vi "Read Module Configuration from Switches JSON.vi"(8 "error in":errorcluster, 11 "switches json file":path) -> (0 "error out":errorcluster, 2 "switches json":string, 3 "topologies":string[](array[string]))   [LabVIEW 2020, in "SLSC Switch Scripting.lvlib"]
uses:
  SLSC Switch Scripting.lvlib
  <vilib>/SLSC_Switch/Get Topologies (Simulate).vi
  <vilib>/SLSC_Switch/SLSC Switch.lvlib
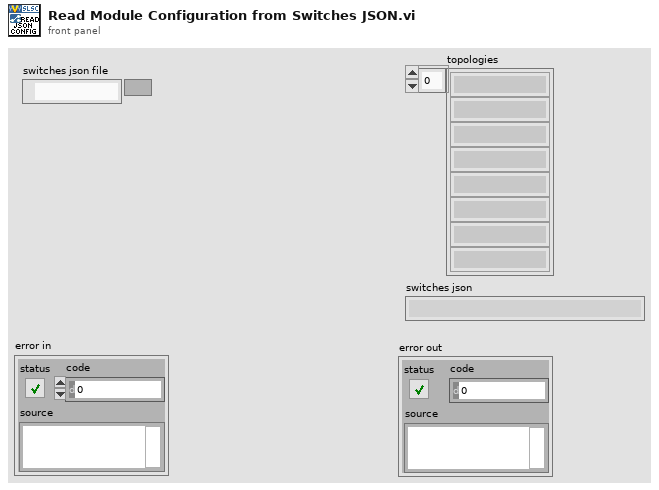
[diagram p1: front panel]
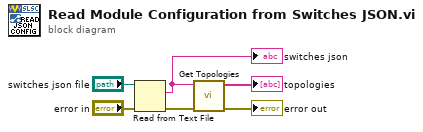
[diagram p0: block diagram]
diagram:
  n1 = Read from Text File(file (use dialog)="switches json file", error in="error in") -> (text=w1:string, error out=w3:errorcluster)  [unwired: 2 in, 2 out]
  "switches json" <- w1
  n2 = call-poly <vilib>:"Get Topologies.vi"("error in (no error)"=w3, "switches json"=w1) -> ("error out"=→"error out":errorcluster, "topologies"=→"topologies":string[])  [unwired: 8 in]
